vi "MDrive_Get_Parameter.vi"(4 "Device Name":string, 6 "Mdrive Mode":T1=enum."Party Mode", 8 "error in":errorcluster, 10 "Get Parameter":T2, 11 "VISA IN":refnum<visa-resource-name>) -> (0 "error out":errorcluster, 1 "Parameter Data Numeric":i32, 2 "Parameter Data String":string, 3 "VISA OUT":refnum<visa-resource-name>)   [LabVIEW 2015]
uses:
  System Control App/Code/Global Variables.vi
  MDrive Mode.ctl
  Get Parameter.ctl
panel:
  # "(Only in Party mode)"
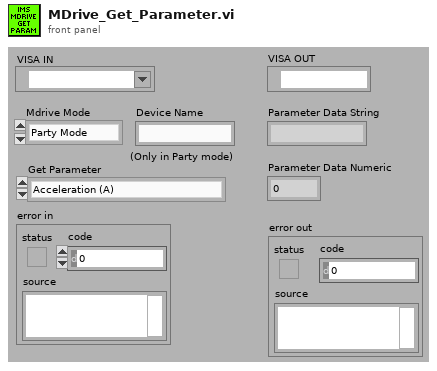
[diagram p1: front panel]
types:
  T1 = typedef "MDrive Mode.ctl" = enum16{"Normal Mode", "Party Mode"}
  T2 = typedef "Get Parameter.ctl" = enum16{"Acceleration (A)", "Baud Rate (BD)", "Busy Flag (BY)", "Counter 1 (C1)", "Counter 2 (C2)", "Check Sum Enable (CK)", "Clock Mode (CM)", "Clock Mode Ratio (CR)", "Clock Mode Out Step Width (CW)", "Deceleration (D)", "Digital Filtering, Input 1 (D1)", "Digital Filtering, Input 2 (D2)", "Digital Filtering, Input 3 (D3)", "Digital Filtering, Input 4 (D4)", "Digital Filtering, Input 5 (D5)", "Digital Filtering, Input 9 (D9)", "Digital Filtering, Input 10 (D10)", "Digital Filtering, Input 11 (D11)", "Digital Filtering, Input 12 (D12)", "Deadband (DB)", "Enable/Disable Drive (DE)", "Device Name (DN)", "End Program Execution (E)", "Encoder Function Enable (EE)", "Encoder Lines (EL)", "Error Flag (EF)", "Error Variable (ER)", "Echo Mode (EM)", "Escape (ES)", "Execute Program at Address (EX)", "Hold Current (HC)", "Hold Current Delay Time (HI)", "Input 1 (I1)", "Input 2 (I2)", "Input 3 (I3)", "Input 4 (I4)", "Input 5 Analog (I5)", "Input 6 Encoder Index (I6)", "Input 9 (I9)", "Input 10 (I10)", "Input 11 (I11)", "Input 12 (I12)", "Input Low Byte (1-4) (IL)", "Input High Byte (9-12) (IH)", "Inputs Total (1-4,9-12) (IN)", "Internal Temperature (IT)", "Jog Enable (JE)", "Limit Stop Mode (LM)", "MicroStepping Select (MS)", "Motor Settling Delay Time (MT)", "Moving Flag (MV)", "Output 1 (O1)", "Output 2 (O2)", "Output 3 (O3)", "Output 4 (O4)", "Output 9 (O9)", "Output 10 (O10)", "Output 11 (O11)", "Output 12 (O12)", "Output High Byte (9-12) (OH)", "Output Low Byte (1-4) (OL)", "Output Total (1-4 and 9-12) (OT)", "Position (P)", "Position Captured at Trip (PC)", "Position Maintenance (PM)", "Part Number (PN)", "Party Mode (PY)", "Register 1 (R1)", "Register 2 (R2)", "Register 3 (R3)", "Register 4 (R4)", "Run Current (RC)", "Serial Number (SN)", "Stall Flag (ST)", "Stall Factor (SF)", "Stall Mode Set (SM)", "User Variables (UV)", "Velocity (V)", "Velocity Changing Flag (VC)", "Velocity Initial (VI)", "Version, Firmware (VR)", "Velocity Maximum (VM)", "Read Input1", "Read Input2"}
  T3 = typedef "Semaphore RefNum" = refnum<k1>
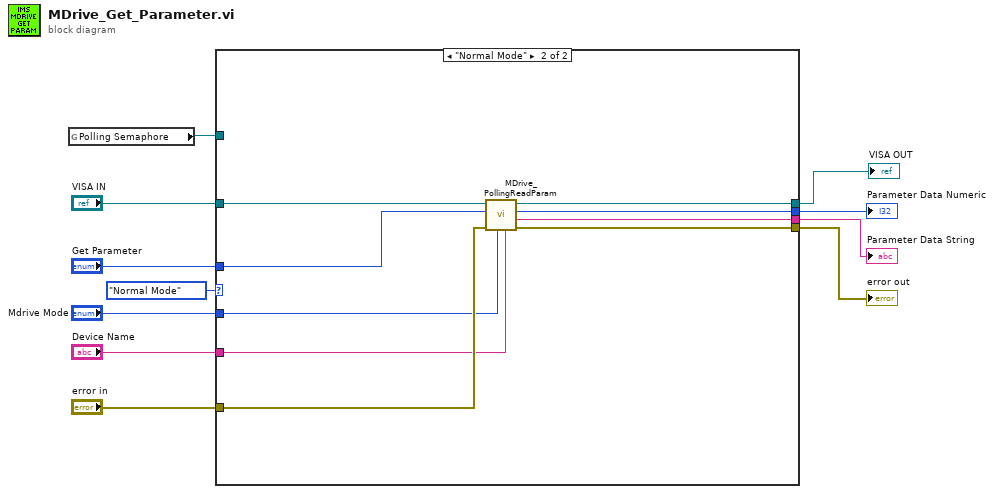
[diagram p0: block diagram]
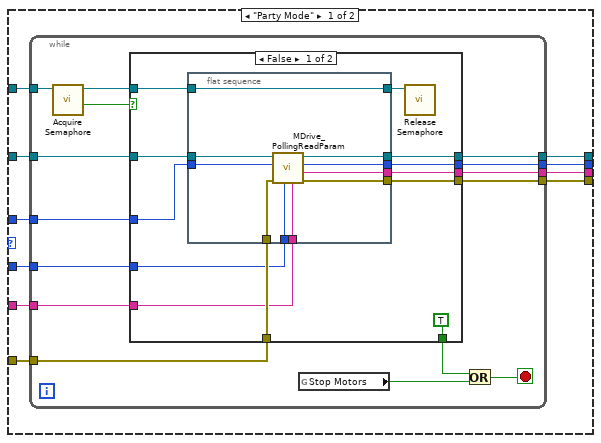
[diagram p2: hidden frame]
diagram:
  n1 = global read "Global Variables.vi" "Polling Semaphore"() -> (w3:T3)
  n2 = case shown="\"Normal Mode\"" MDrive_Mode."Normal Mode" ("Mdrive Mode") {
    tunnel: [w21 w69] -> w11
    tunnel: "VISA IN" -> [w20 w68]
    tunnel: "error in" -> [w19 w67]
    tunnel: "Get Parameter" -> [w18 w66]
    tunnel: [w17 w65] -> w7
    tunnel: [w16 w64] -> w6
    tunnel: [w15 w63] -> w5
    tunnel: "Device Name" -> [w14 w62]
    tunnel: "Mdrive Mode" -> [w13 w61]
    tunnel: w3 -> [w12 _]
    frame "Party Mode" {
      n3 = while {
        tunnel: [w36] -> w21
        tunnel: w20 -> [w35]
        tunnel: w19 -> [w34]
        tunnel: w18 -> [w33]
        tunnel: [w32] -> w17
        tunnel: [w31] -> w16
        tunnel: [w30] -> w15
        tunnel: w14 -> [w29]
        tunnel: w13 -> [w28]
        tunnel: w12 -> [w27]
        stop <- w24 stop-if-true
        n4 = call <vilib>:"Acquire Semaphore.vi"("semaphore"=w27) -> ("timed out"=w26:bool, "semaphore out"=w25:T3)  [unwired: 4 in, 1 out]
        n5 = case shown="False" w26 {
          tunnel: [w48 w60] -> w36
          tunnel: w35 -> [w47 w60]
          tunnel: w34 -> [w46 w59]
          tunnel: w33 -> [w45 _]
          tunnel: [w44 _] -> w32
          tunnel: [w43 _] -> w31
          tunnel: [w42 w59] -> w30
          tunnel: w29 -> [w41 _]
          tunnel: w28 -> [w40 _]
          tunnel: w25 -> [w39 _]
          tunnel: [TRUE ("timed out") _] -> w23
          frame False {
            n6 = flat-sequence {
              tunnel: [w58] -> w48
              tunnel: w47 -> [w57]
              tunnel: w46 -> [w56]
              tunnel: w45 -> [w55]
              tunnel: [w54] -> w44
              tunnel: [w53] -> w43
              tunnel: [w52] -> w42
              tunnel: w41 -> [w51]
              tunnel: w40 -> [w50]
              tunnel: [w49] -> w38
              tunnel: w39 -> [w49]
              frame #0 {
                n7 = call "MDrive_PollingReadParam.vi"("Device Name"=w51, "Mdrive Mode"=w50, "error in (no error)"=w56, "Get Parameter"=w55, "VISA Refnum in"=w57) -> ("error out"=w52:errorcluster, "String"=w54:string, "Value"=w53:i32, "VISA Refnum out"=w58:refnum<visa-resource-name>)  [unwired: 3 in]
              }
            }
            n8 = call <vilib>:"Release Semaphore.vi"("semaphore"=w38) -> ()  [unwired: 5 in, 2 out]
          }
          frame True {
          }
        }
        n9 = global read "Global Variables.vi" "Stop Motors"() -> (w22:bool)
        n10 = Or(x=w23, y=w22) -> (x .or. y?=w24:bool)
      }
    }
    frame "Normal Mode" {
      n11 = call "MDrive_PollingReadParam.vi"("Device Name"=w62, "Mdrive Mode"=w61, "error in (no error)"=w67, "Get Parameter"=w66, "VISA Refnum in"=w68) -> ("error out"=w63:errorcluster, "String"=w65:string, "Value"=w64:i32, "VISA Refnum out"=w69:refnum<visa-resource-name>)  [unwired: 3 in]
    }
  }
  "error out" <- w5
  "VISA OUT" <- w11
  "Parameter Data String" <- w7
  "Parameter Data Numeric" <- w6
